vi "Pracowania_6_global.vi"() -> ()   [LabVIEW 2019]
panel:
  in  "stop":bool
  out "tablica bitow":bool[](array[boolean])
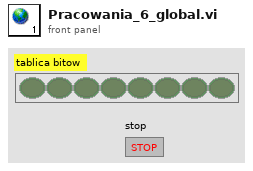
[diagram p1: front panel]
diagram:
